vi "Execute received commands.vi"(8 "error in (no error)":errorcluster, 10 "WCM_state":bool=TRUE, 11 "Control-Client in":refnum<class "Control-Client.lvclass">) -> (0 "error out":errorcluster, 3 "Control-Client out":refnum<class "Control-Client.lvclass">)   [LabVIEW 2018, in "Control-Client.lvclass"]
uses:
  Control-Client.lvclass
  C:/Users/Sergey Denisov/Documents/REPS/TRANCON/Classes/GeneralFunctionality/GeneralFunctionality.lvclass
  dependecies/ControlsVIs/Clusters-def/Det-Reply-to-Read.ctl
  dependecies/ControlsVIs/Clusters-def/Def_signals_from_DET.ctl
  dependecies/ControlsVIs/Clusters-def/Message types.ctl
  dependecies/ControlsVIs/Clusters-def/Standard Command.ctl
  Control-Client.lvclass/Control-Client.ctl
  dependecies/ControlsVIs/Clusters-def/ProtypeCommand-CommandUnknown.ctl
  <vilib>/NI/STM/TCP/TCP Connection Info.ctl
  <vilib>/NI/STM/SubVIs/MetaDataElement.ctl
  dependecies/ControlsVIs/Clusters-def/Commands-CLIENT.ctl
  dependecies/ControlsVIs/Clusters-def/DLMovedAxis-Com.ctl
  dependecies/XControls/CellsDL/ControlDL.xctl
  dependecies/ControlsVIs/Clusters-def/OSc-Reply-Read.ctl
  dependecies/ControlsVIs/Clusters-def/CONTROL-Reply-Allconnect.ctl
  dependecies/ControlsVIs/Clusters-def/ProtypeCommand-DAQmxReply.ctl
  dependecies/ControlsVIs/Clusters-def/DAQmx-ELYSE_pulse_counter.ctl
  dependecies/ControlsVIs/Clusters-def/DAQmx-ELYSE_PumpSpeed.ctl
  controls/Gauge_pump/Gauge_pump.xctl
  dependecies/average-2Darray-SD_double.vi
  Message/Message.lvclass
  <vilib>/NI/STM/NI STM.lvlib
  Control-Server/Control-Server.lvclass
  Delay Line/DelayLine.lvclass
  DAQmxTasks/DAQmxTaskContainer_General/DAQmxTaksContainer_General.lvclass
  Oscilloscope/Oscilloscope.lvclass
  GeneralFunctionality/GeneralFunctionality.lvclass
  Detector/Detector.lvclass
panel:
  in  "?":T1
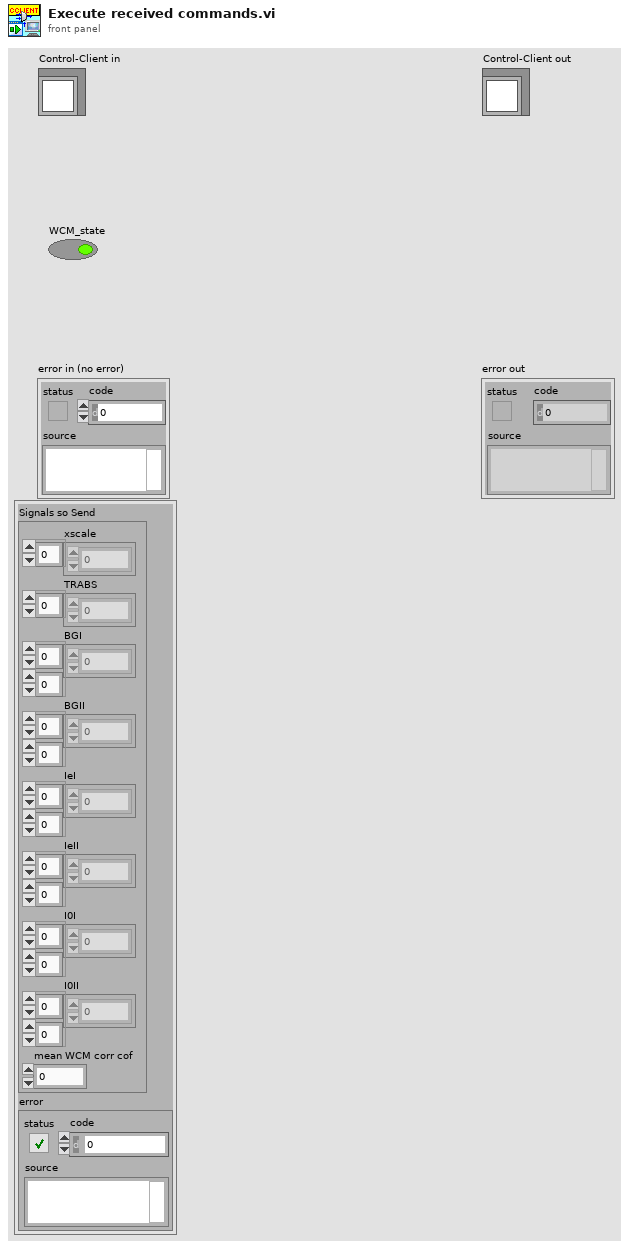
[diagram p1: front panel]
types:
  T1 = typedef "Detector.lvclass/Det-Reply-to-Read.ctl" = cluster{"Signals so Send":T2, "error":errorcluster}
  T2 = typedef "Detector.lvclass/Def_signals_from_DET.ctl" = cluster{"xscale":sgl[], "TRABS":sgl[], "BGI":sgl[][], "BGII":sgl[][], "IeI":sgl[][], "IeII":sgl[][], "I0I":sgl[][], "I0II":sgl[][], "mean WCM corr cof":dbl}
  T3 = typedef "Message types.ctl" = string
  T4 = typedef "Standard Command.ctl" = cluster{"command":string, "data":variant}
  T5 = typedef "ProtypeCommand-CommandUnknown.ctl" = cluster{"error in (no error)":errorcluster}
  T6 = typedef "Control-Client.lvclass/Commands-CLIENT.ctl" = string
  T7 = typedef "NI STM.lvlib/TCP Connection Info.ctl" = cluster{"connection ID":refnum<k5>, "meta data":T8[]}
  T8 = typedef "NI STM.lvlib/MetaDataElement.ctl" = string
  T9 = typedef "DelayLine.lvclass/DLMovedAxis-Com.ctl" = cluster{"axis":i32, "what was asked":dbl, "where is is now":dbl, "Moved":bool, "error in (no error)":errorcluster}
  T10 = typedef "Oscilloscope.lvclass/OSc-Reply-Read.ctl" = cluster{"Data":waveform(dbl)[], "Channels":u16[], "error":errorcluster}
  T11 = typedef "Control-Server.lvclass/CONTROL-Reply-Allconnect.ctl" = cluster{"On/Off":bool, "error":errorcluster}
  T12 = typedef "ProtypeCommand-DAQmxReply.ctl" = cluster{"On/Off":bool, "error out":errorcluster}
  T13 = enum8{"Enabled", "Disabled", "Disabled and Grayed Out"}
  T14 = typedef "DAQmxTaksContainer_General.lvclass/DAQmx-ELYSE_pulse_counter.ctl" = cluster{"# counts":dbl}
  T15 = cluster{"Data":dbl, "direction":bool, "start/stop":bool}
  T16 = typedef "DAQmxTaksContainer_General.lvclass/DAQmx-ELYSE_PumpSpeed.ctl" = cluster{"speed, rpm":dbl}
  T17 = typedef "Control-Client.lvclass/Controls-with-permissions_CLIENT.ctl" = cluster{"Server ON/OFF":refnum<vi>, "Detector connect":refnum<vi>, "DL connect":refnum<vi>, "DAQmx connect":refnum<vi>, "All connect":refnum<vi>, "Start measurement":refnum<vi>, "Move Crystal":refnum<vi>, "Relay key heater":refnum<vi>, "Laser Shutter":refnum<vi>, "Accelerator Shutter":refnum<vi>, "Power":refnum<vi>, "Unlock":refnum<vi>, "RT":refnum<vi>, "Faraday Cup":refnum<vi>, "Osc connect":refnum<vi>, "ELYSE pulses":refnum<vi>, "Cells":refnum<vi>, "Pump":refnum<vi>, "# par point":refnum<vi>, "Alarm":refnum<vi>, "oscilloscopeRead":refnum<vi>, "WCM_state":refnum<vi>, "ControlDL":refnum<vi>}
  T18 = typedef "graphs_TR.ctl" = cluster{"TR SC":refnum<vi>, "TR OD":refnum<vi>, "Raw data":refnum<vi>, "Raw data BG":refnum<vi>}
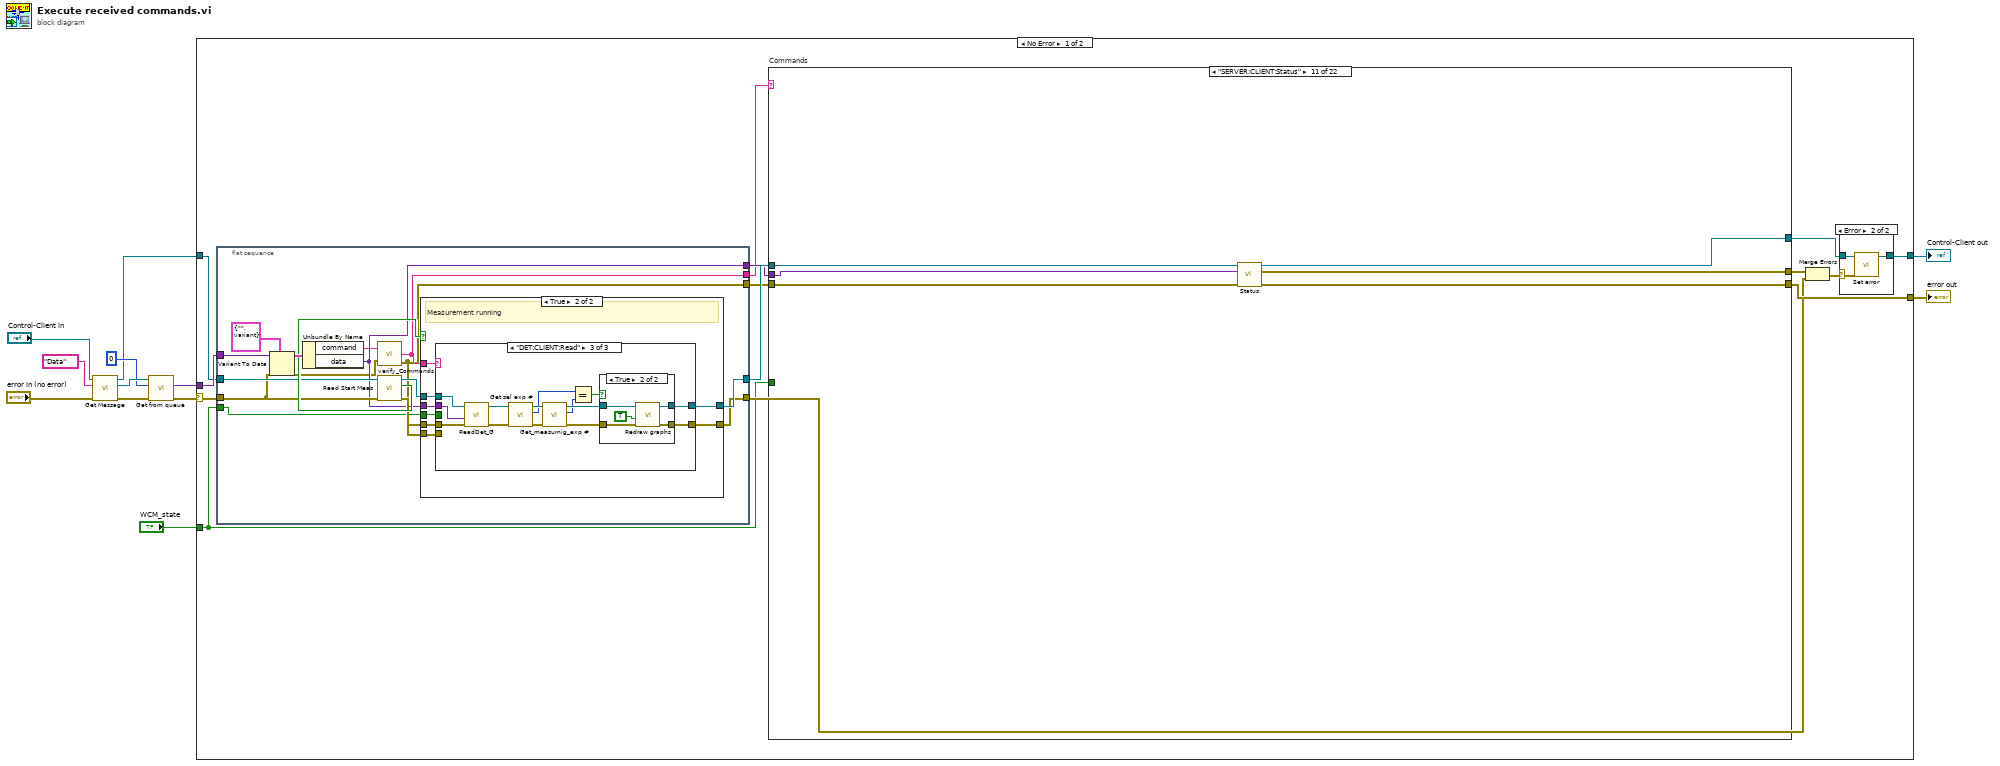
[diagram p0: block diagram]
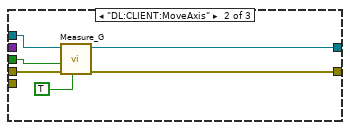
[diagram p5: hidden frame]
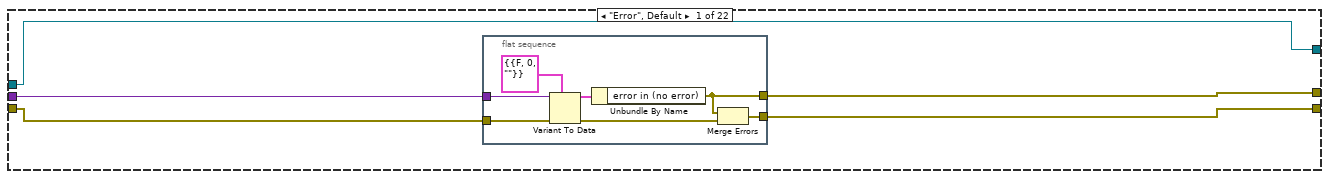
[diagram p7: hidden frame]
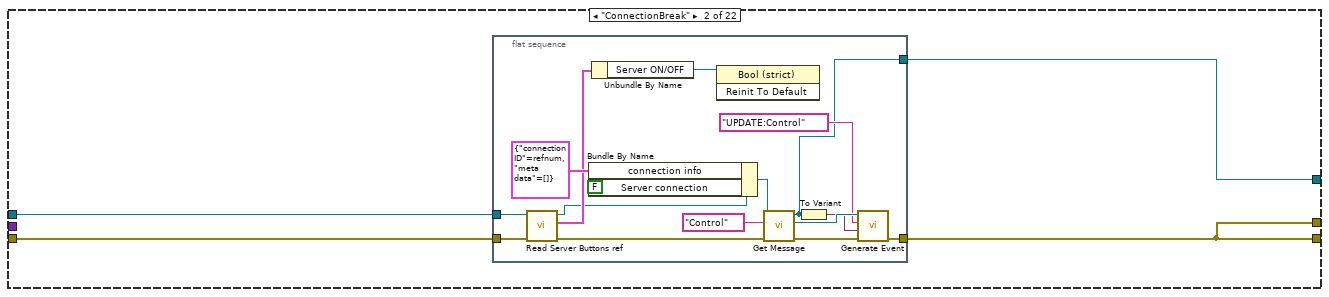
[diagram p8: hidden frame]
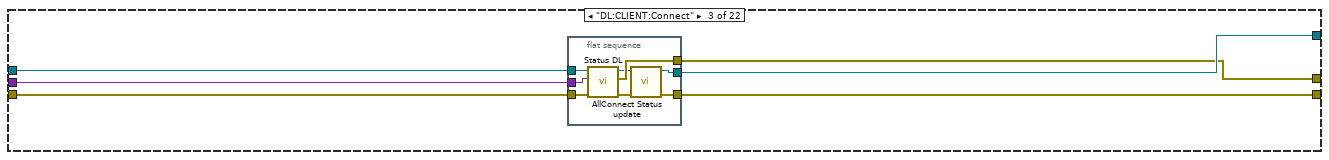
[diagram p9: hidden frame]
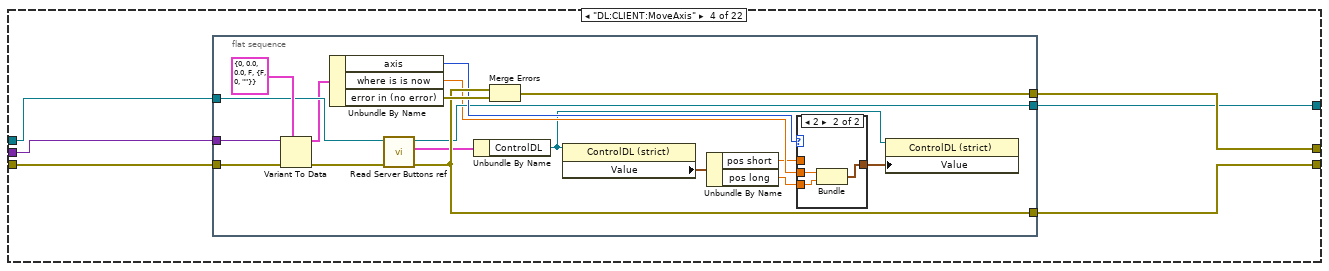
[diagram p10: hidden frame]
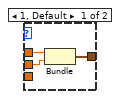
[diagram p11: hidden frame]
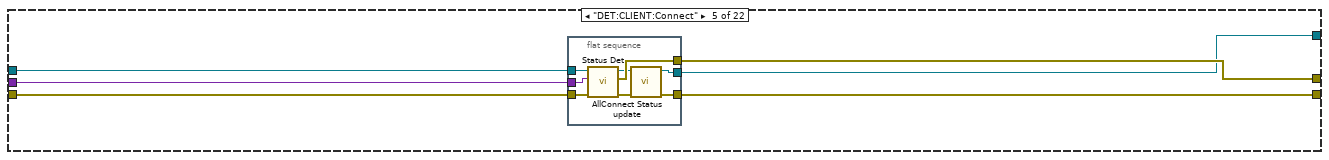
[diagram p12: hidden frame]
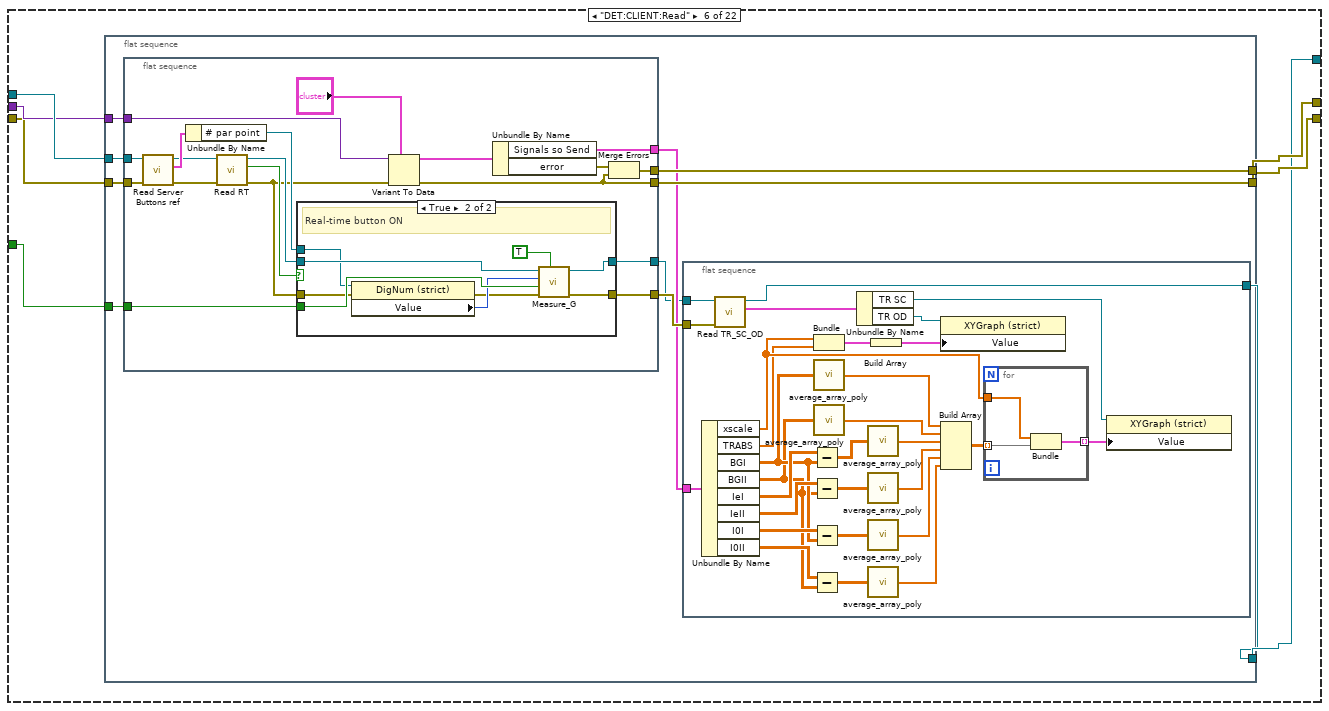
[diagram p13: hidden frame]
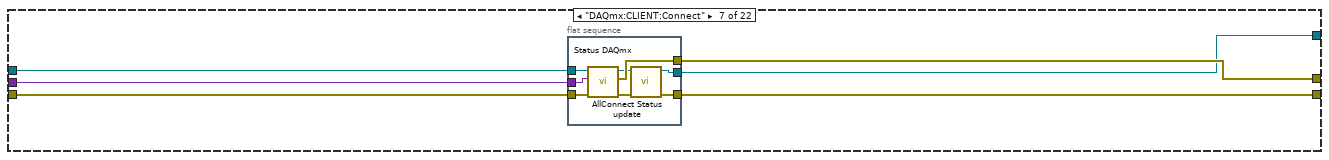
[diagram p15: hidden frame]
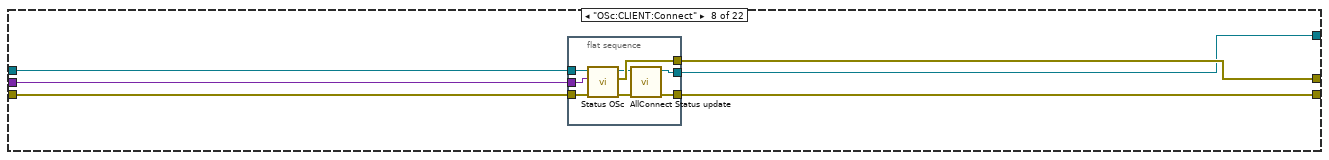
[diagram p16: hidden frame]
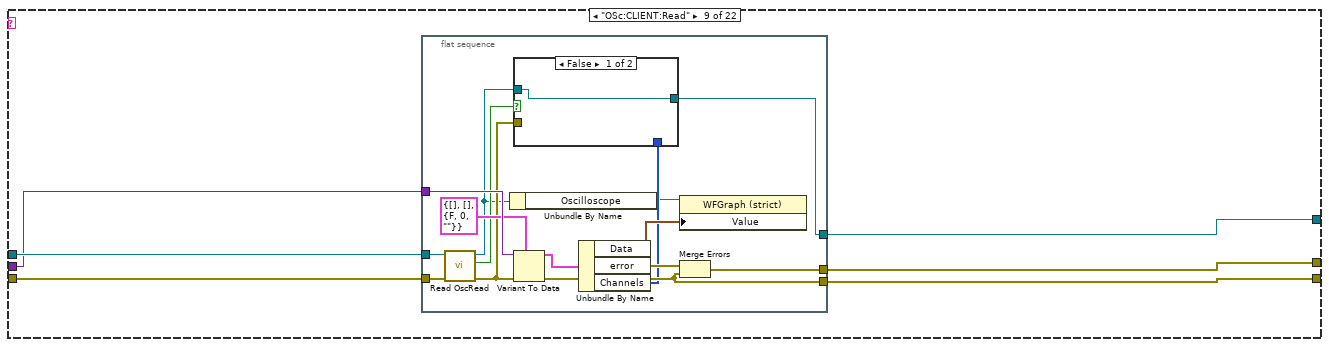
[diagram p17: hidden frame]
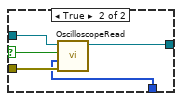
[diagram p18: hidden frame]
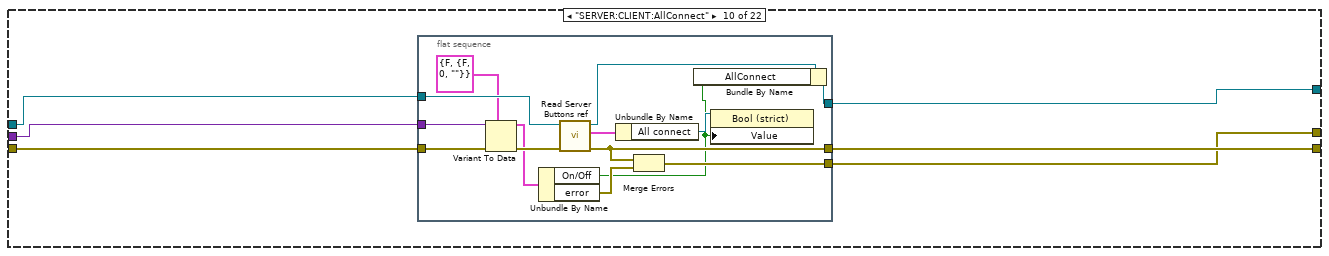
[diagram p19: hidden frame]
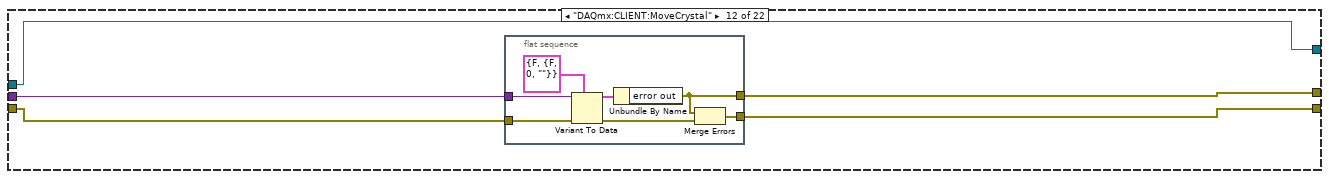
[diagram p20: hidden frame]
diagram:
  n1 = call "Get Message.vi"("error in (no error)"="error in (no error)", "Message type"=T3 "Data", "GeneralFunctionality en entrée"="Control-Client in") -> ("error out"=w6:errorcluster, "Message.lvclass"=w7:refnum<class "Message.lvclass">, "GeneralFunctionality en sortie"=w1:refnum<class "Control-Client.lvclass">)  [unwired: 6 in]
  n2 = call "Get from queue.vi"("error in (no error)"=w6, "timeout in ms (-1)"=0, "Message in"=w7) -> ("error out"=w5:errorcluster, "Data"=w4:variant)  [unwired: 5 in, 2 out]
  n3 = case shown="No Error" w5 {
    selector: w5 -> [w21 w531]
    tunnel: w4 -> [w26 _]
    tunnel: w1 -> [w22 w530]
    tunnel: [w25 w531] -> w11
    tunnel: [w23 w530] -> w9
    tunnel: "WCM_state" -> [w14 _]
    frame No Error {
      n4 = flat-sequence {
        tunnel: w26 -> [w46]
        tunnel: w22 -> [w42]
        tunnel: w21 -> [w41]
        tunnel: [w38] -> w19
        tunnel: [w37] -> w18
        tunnel: [w34] -> w17
        tunnel: [w33] -> w16
        tunnel: [w32] -> w15
        tunnel: w14 -> [w31]
        frame #0 {
          n5 = Variant To Data(error in=w41, type=T4 {"command"="", "data"=variant} ("input cluster"), Variant=w46) -> (data=w44:T4, error out=w36:errorcluster)
          n6 = Unbundle By Name(w44) -> ("command"=w35:string, "data"=w37:variant)
          n7 = call "verify_Commands.vi"("Command"=w35, "error in"=w36) -> ("Command out"=w34:string, "error out"=w33:errorcluster)  [unwired: 1 out]
          n8 = call "Read Start Meas.vi"("error in (no error)"=w41, "Control-Client in"=w42) -> ("error out"=w40:errorcluster, "Start Meas"=w43:bool, "Control-Client out"=w39:refnum<class "Control-Client.lvclass">)  [unwired: 7 in]
          n9 = case shown="True" w43 {
            tunnel: w34 -> [_ w56]
            tunnel: w40 -> [w48 w55]
            tunnel: [w48 w52] -> w32
            tunnel: w39 -> [w47 w54]
            tunnel: [w47 w53] -> w38
            tunnel: w37 -> [_ w51]
            tunnel: w33 -> [_ w50]
            tunnel: w31 -> [_ w49]
            frame False {
              # "Measurement not running"
            }
            frame True {
              # "Measurement running"
              n10 = case shown="\"DET:CLIENT:Read\"" w56 {
                tunnel: w55 -> [_ w61 w78]
                tunnel: [w57 w64 w76] -> w52
                tunnel: w54 -> [w58 w62 w77]
                tunnel: [w58 w63 w75] -> w53
                tunnel: w51 -> [_ _ w74]
                tunnel: w50 -> [w57 _ _]
                tunnel: w49 -> [_ w60 _]
                frame "Error", Default {
                }
                frame "DL:CLIENT:MoveAxis" {
                  n11 = call "Measure_G.vi"("Internal"=TRUE ("Inernal"), "error in (no error)"=w61, "WCM_correction"=w60, "Control-Client in"=w62) -> ("error out"=w64:errorcluster, "Control-Client out"=w63:refnum<class "Control-Client.lvclass">)  [unwired: 6 in]
                }
                frame "DET:CLIENT:Read" {
                  n12 = call "ReadDet_G.vi"("error in (no error)"=w78, "data"=w74, "Control-Client in"=w77) -> ("error out"=w69:errorcluster, "Control-Client out"=w72:refnum<class "Control-Client.lvclass">)  [unwired: 7 in]
                  n13 = call "Get sel exp #.vi"("error in (no error)"=w69, "Control-Client in"=w72) -> ("error out"=w70:errorcluster, "Exp sel #"=w67:i32, "Control-Client out"=w73:refnum<class "Control-Client.lvclass">)  [unwired: 7 in]
                  n14 = call "Get_measurnig_exp #.vi"("error in (no error)"=w70, "Control-Client in"=w73) -> ("error out"=w68:errorcluster, "Exp measuring #"=w66:i32, "Control-Client out"=w71:refnum<class "Control-Client.lvclass">)  [unwired: 7 in]
                  n15 = Equal?(x=w67, y=w66) -> (x = y?=w65:bool)
                  n16 = case shown="True" w65 {
                    tunnel: [w80 w85] -> w76
                    tunnel: [w79 w84] -> w75
                    tunnel: w71 -> [w79 w82]
                    tunnel: w68 -> [w80 w81]
                    frame False {
                    }
                    frame True {
                      n17 = call "Redraw graphs.vi"("error in (no error)"=w81, "Selected exp"=TRUE, "Control-Client in"=w82) -> ("error out"=w85:errorcluster, "Control-Client out"=w84:refnum<class "Control-Client.lvclass">)  [unwired: 7 in]
                    }
                  }
                }
              }
            }
          }
        }
      }
      n18 = case "Commands" shown="\"SERVER:CLIENT:Status\"" w17 {
        tunnel: w18 -> [w90 _ w123 w137 w167 w181 w260 w274 w287 w315 w335 w340 w353 w370 w389 w410 w431 w450 w467 w487 w506 w522]
        tunnel: w19 -> [w89 w99 w122 w135 w166 w182 w259 w273 w288 w314 w334 w338 w352 w372 w391 w409 w432 w451 w468 w488 w507 w523]
        tunnel: w16 -> [w87 w98 w121 w136 w165 w177 w258 w272 w283 w313 w333 w337 w351 w371 w390 w408 w433 w452 w469 w483 w502 w518]
        tunnel: [w86 w100 w119 w133 w162 w180 w255 w269 w286 w311 w331 w336 w350 w369 w386 w407 w430 w449 w466 w486 w505 w521] -> w25
        tunnel: [w89 w101 w120 w132 w163 w178 w256 w270 w284 w312 w332 w338 w348 w367 w388 w405 w428 w447 w464 w484 w503 w519] -> w24
        tunnel: [w88 w100 w118 w134 w164 w179 w257 w271 w285 w310 w330 w339 w349 w368 w387 w406 w429 w448 w465 w485 w504 w520] -> w20
        tunnel: w14 -> [_ _ _ _ _ w176 _ _ _ _ _ _ _ _ _ _ _ _ _ _ _ _]
        frame "Error", Default {
          n19 = flat-sequence {
            tunnel: w90 -> [w97]
            tunnel: [w93] -> w88
            tunnel: w87 -> [w94]
            tunnel: [w91] -> w86
            frame #0 {
              n20 = Variant To Data(error in=w94, type=T5 {"error in (no error)"={"status"=FALSE, "code"=0, "source"=""}} ("cluster"), Variant=w97) -> (data=w95:T5, error out=w92:errorcluster)
              n21 = Unbundle By Name(w95) -> ("error in (no error)"=w93:errorcluster)
              n22 = Merge Errors(w93, w92) -> (w91:errorcluster)
            }
          }
        }
        frame "ConnectionBreak" {
          n23 = flat-sequence {
            tunnel: [w102] -> w101
            tunnel: [w110] -> w100
            tunnel: w99 -> [w109]
            tunnel: w98 -> [w108]
            frame #0 {
              n24 = call "Read Server Buttons ref.vi"("error in (no error)"=w108, "Control-Client in"=w109) -> ("error out"=w107:errorcluster, "Server Buttons ref"=w106:T17, "Control-Client out"=w103:refnum<class "Control-Client.lvclass">)  [unwired: 7 in]
              n25 = Bundle By Name(cluster=w103, "connection info"=T7 {"connection ID"=refnum, "meta data"=[]}, "Server connection"=FALSE) -> (w111:refnum<class "Control-Client.lvclass">)
              n26 = Unbundle By Name(w106) -> ("Server ON/OFF"=w104:refnum<vi>)
              n27 = invoke class="Bool (strict)" method="Reinit To Default"(reference=w104) -> ()  [unwired: 2 in, 3 out]
              n28 = call "Get Message.vi"("error in (no error)"=w107, "Message type"=T3 "Control", "GeneralFunctionality en entrée"=w111) -> ("error out"=w115:errorcluster, "Message.lvclass"=w114:refnum<class "Message.lvclass">, "GeneralFunctionality en sortie"=w102:refnum<class "Control-Client.lvclass">)  [unwired: 6 in]
              n29 = To Variant(anything=w102) -> (Variant=w112:variant)
              n30 = call "Generate Event.vi"("error in (no error)"=w115, "Data"=w112, "Command"=T6 "UPDATE:Control" ("Commands-Client"), "Message en entrée"=w114) -> ("error out"=w110:errorcluster)  [unwired: 6 in, 1 out]
            }
          }
        }
        frame "DL:CLIENT:Connect" {
          n31 = flat-sequence {
            tunnel: w123 -> [w131]
            tunnel: w122 -> [w130]
            tunnel: w121 -> [w129]
            tunnel: [w126] -> w120
            tunnel: [w125] -> w119
            tunnel: [w128] -> w118
            frame #0 {
              n32 = call "Status DL.vi"("error in (no error)"=w129, "data"=w131, "Control-Client in"=w130) -> ("error out"=w124:errorcluster, "error IO"=w128:errorcluster, "Control-Client out"=w127:refnum<class "Control-Client.lvclass">)  [unwired: 6 in]
              n33 = call "AllConnect Status update.vi"("error in (no error)"=w124, "Control-Client in"=w127) -> ("error out"=w125:errorcluster, "Control-Client out"=w126:refnum<class "Control-Client.lvclass">)  [unwired: 8 in]
            }
          }
        }
        frame "DL:CLIENT:MoveAxis" {
          n34 = flat-sequence {
            tunnel: w137 -> [w155]
            tunnel: w136 -> [w154]
            tunnel: w135 -> [w151]
            tunnel: [w148] -> w134
            tunnel: [w147] -> w133
            tunnel: [w145] -> w132
            frame #0 {
              n35 = Variant To Data(error in=w154, type=T9 {"axis"=0, "what was asked"=0.0, "where is is now"=0.0, "Moved"=FALSE, "error in (no error)"={"status"=FALSE, "code"=0, "source"=""}} ("cluster"), Variant=w155) -> (data=w150:T9, error out=w152:errorcluster)
              n36 = Unbundle By Name(w150) -> ("axis"=w146:i32, "where is is now"=w144:dbl, "error in (no error)"=w149:errorcluster)
              n37 = call "Read Server Buttons ref.vi"("error in (no error)"=w152, "Control-Client in"=w151) -> ("error out"=w147:errorcluster, "Server Buttons ref"=w142:T17, "Control-Client out"=w145:refnum<class "Control-Client.lvclass">)  [unwired: 7 in]
              n38 = Unbundle By Name(w142) -> ("ControlDL"=w139:refnum<vi>)
              n39 = Merge Errors(w147, w149) -> (w148:errorcluster)
              n40 = property class="ControlDL (strict)"(reference=w139) -> ("Value"=w141:cluster{"pos short":dbl, "pos long":dbl})  [unwired: 1 in, 2 out]
              n41 = Unbundle By Name(w141) -> ("pos short"=w140:dbl, "pos long"=w138:dbl)
              n42 = case shown="2" w146 {
                tunnel: w144 -> [w158 w161]
                tunnel: [w157 w159] -> w143
                tunnel: w140 -> [w156 _]
                tunnel: w138 -> [_ w160]
                frame 1, Default {
                  n43 = Bundle("pos short"=w156, "where is is now"=w158) -> (w157:cluster{"pos short":dbl, "where is is now":dbl})  [unwired: 1 in]
                }
                frame 2 {
                  n44 = Bundle("where is is now"=w161, "pos long"=w160) -> (w159:cluster{"where is is now":dbl, "pos long":dbl})  [unwired: 1 in]
                }
              }
              n45 = property class="ControlDL (strict)"(reference=w139, "Value"=w143) -> ()  [unwired: 1 in, 2 out]
            }
          }
        }
        frame "DET:CLIENT:Connect" {
          n46 = flat-sequence {
            tunnel: w167 -> [w175]
            tunnel: w166 -> [w174]
            tunnel: w165 -> [w173]
            tunnel: [w172] -> w164
            tunnel: [w170] -> w163
            tunnel: [w168] -> w162
            frame #0 {
              n47 = call "Status Det.vi"("error in (no error)"=w173, "data"=w175, "Control-Client in"=w174) -> ("error out"=w169:errorcluster, "error IO"=w172:errorcluster, "Control-Client out"=w171:refnum<class "Control-Client.lvclass">)  [unwired: 6 in]
              n48 = call "AllConnect Status update.vi"("error in (no error)"=w169, "Control-Client in"=w171) -> ("error out"=w168:errorcluster, "Control-Client out"=w170:refnum<class "Control-Client.lvclass">)  [unwired: 8 in]
            }
          }
        }
        frame "DET:CLIENT:Read" {
          n49 = flat-sequence {
            tunnel: w182 -> [w189]
            tunnel: w181 -> [w192]
            tunnel: [w191] -> w180
            tunnel: [w190] -> w179
            tunnel: [w183] -> w178
            tunnel: w177 -> [w188]
            tunnel: w176 -> [w185]
            frame #0 {
              n50 = flat-sequence {
                tunnel: w192 -> [w211]
                tunnel: [w210] -> w191
                tunnel: [w209] -> w190
                tunnel: w189 -> [w205]
                tunnel: w188 -> [w199]
                tunnel: [w195] -> w187
                tunnel: [w201] -> w186
                tunnel: w185 -> [w200]
                tunnel: [w197] -> w184
                frame #0 {
                  n51 = call "Read Server Buttons ref.vi"("error in (no error)"=w199, "Control-Client in"=w205) -> ("error out"=w193:errorcluster, "Server Buttons ref"=w204:T17, "Control-Client out"=w194:refnum<class "Control-Client.lvclass">)  [unwired: 7 in]
                  n52 = Unbundle By Name(w204) -> ("# par point"=w203:refnum<vi>)
                  n53 = call "Read RT.vi"("error in (no error)"=w193, "Control-Client in"=w194) -> ("error out"=w196:errorcluster, "RT"=w202:bool, "Control-Client out"=w198:refnum<class "Control-Client.lvclass">)  [unwired: 7 in]
                  n54 = case shown="True" w202 {
                    tunnel: w198 -> [w213 w222]
                    tunnel: w196 -> [w212 w217]
                    tunnel: w203 -> [_ w219]
                    tunnel: w200 -> [_ w221]
                    tunnel: [w213 w215] -> w197
                    tunnel: [w212 w214] -> w195
                    frame False {
                    }
                    frame True {
                      # "Real-time button ON"
                      n55 = property class="DigNum (strict)"(reference=w219, error in=w217) -> (error out=w216:errorcluster, "Value"=w218:i32)  [unwired: 1 out]
                      n56 = call "Measure_G.vi"("All"=TRUE, "error in (no error)"=w216, "WCM_correction"=w221, "# scans"=w218, "Control-Client in"=w222) -> ("error out"=w214:errorcluster, "Control-Client out"=w215:refnum<class "Control-Client.lvclass">)  [unwired: 5 in]
                    }
                  }
                  n57 = Variant To Data(error in=w196, type="?", Variant=w211) -> (data=w207:T1, error out=w210:errorcluster)
                  n58 = Unbundle By Name(w207) -> ("Signals so Send"=w201:T2, "error"=w206:errorcluster)
                  n59 = Merge Errors(w206, w210) -> (w209:errorcluster)
                }
              }
              n60 = flat-sequence {
                tunnel: w187 -> [w236]
                tunnel: w186 -> [w246]
                tunnel: w184 -> [w234]
                tunnel: [w233] -> w183
                frame #0 {
                  n61 = Unbundle By Name(w246) -> ("xscale"=w248:sgl[], "TRABS"=w247:sgl[], "BGI"=w224:sgl[][], "BGII"=w223:sgl[][], "IeI"=w232:sgl[][], "IeII"=w230:sgl[][], "I0I"=w228:sgl[][], "I0II"=w225:sgl[][])
                  n62 = call "Read TR_SC_OD.vi"("error in (no error)"=w236, "Control-Client en entrée"=w234) -> ("TR_SC_OD"=w235:T18, "Control-Client en sortie"=w233:refnum<class "Control-Client.lvclass">)  [unwired: 7 in, 1 out]
                  n63 = Subtract(x=w232, y=w224) -> (x-y=w231:sgl[][])
                  n64 = Subtract(x=w230, y=w223) -> (x-y=w229:sgl[][])
                  n65 = Subtract(x=w228, y=w224) -> (x-y=w227:sgl[][])
                  n66 = Subtract(x=w225, y=w223) -> (x-y=w226:sgl[][])
                  n67 = Bundle("xscale"=w248, "TRABS"=w247) -> (w249:cluster{"xscale":sgl[], "TRABS":sgl[]})  [unwired: 1 in]
                  n68 = call-poly "average_array_poly.vi"("2D array"=w224) -> ("out array"=w242:dbl[])
                  n69 = call-poly "average_array_poly.vi"("2D array"=w223) -> ("out array"=w241:dbl[])
                  n70 = Unbundle By Name(w235) -> ("TR SC"=w251:refnum<vi>, "TR OD"=w250:refnum<vi>)
                  n71 = call-poly "average_array_poly.vi"("2D array"=w231) -> ("out array"=w240:dbl[])
                  n72 = call-poly "average_array_poly.vi"("2D array"=w229) -> ("out array"=w239:dbl[])
                  n73 = call-poly "average_array_poly.vi"("2D array"=w227) -> ("out array"=w238:dbl[])
                  n74 = call-poly "average_array_poly.vi"("2D array"=w226) -> ("out array"=w237:dbl[])
                  n75 = Build Array(w249) -> (w243:cluster{"xscale":sgl[], "TRABS":sgl[]}[])
                  n76 = property class="XYGraph (strict)"(reference=w250, "Value"=w243) -> ()  [unwired: 1 in, 2 out]
                  n77 = Build Array(w242, w241, w240, w239, w238, w237) -> (w245:dbl[][])
                  n78 = for {
                    tunnel: [w254] -> w244 mode=indexing
                    tunnel: w248 -> [w253]
                    tunnel: w245 -> [w252] mode=indexing
                    n79 = Bundle("xscale"=w253, w252) -> (w254:cluster{"xscale":sgl[], dbl[]})  [unwired: 1 in]
                  }
                  n80 = property class="XYGraph (strict)"(reference=w251, "Value"=w244) -> ()  [unwired: 1 in, 2 out]
                }
              }
            }
          }
        }
        frame "DAQmx:CLIENT:Connect" {
          n81 = flat-sequence {
            tunnel: w260 -> [w268]
            tunnel: w259 -> [w267]
            tunnel: w258 -> [w266]
            tunnel: [w265] -> w257
            tunnel: [w262] -> w256
            tunnel: [w261] -> w255
            frame #0 {
              n82 = call "Status DAQmx.vi"("error in (no error)"=w266, "data"=w268, "Control-Client in"=w267) -> ("error out"=w263:errorcluster, "error IO"=w265:errorcluster, "Control-Client out"=w264:refnum<class "Control-Client.lvclass">)  [unwired: 6 in]
              n83 = call "AllConnect Status update.vi"("error in (no error)"=w263, "Control-Client in"=w264) -> ("error out"=w261:errorcluster, "Control-Client out"=w262:refnum<class "Control-Client.lvclass">)  [unwired: 8 in]
            }
          }
        }
        frame "OSc:CLIENT:Connect" {
          n84 = flat-sequence {
            tunnel: w274 -> [w282]
            tunnel: w273 -> [w281]
            tunnel: w272 -> [w280]
            tunnel: [w279] -> w271
            tunnel: [w276] -> w270
            tunnel: [w275] -> w269
            frame #0 {
              n85 = call "Status OSc.vi"("error in (no error)"=w280, "data"=w282, "Control-Client in"=w281) -> ("error out"=w277:errorcluster, "error IO"=w279:errorcluster, "Control-Client out"=w278:refnum<class "Control-Client.lvclass">)  [unwired: 6 in]
              n86 = call "AllConnect Status update.vi"("error in (no error)"=w277, "Control-Client in"=w278) -> ("error out"=w275:errorcluster, "Control-Client out"=w276:refnum<class "Control-Client.lvclass">)  [unwired: 8 in]
            }
          }
        }
        frame "OSc:CLIENT:Read" {
          n87 = flat-sequence {
            tunnel: w288 -> [w296]
            tunnel: w287 -> [w303]
            tunnel: [w301] -> w286
            tunnel: [w300] -> w285
            tunnel: [w289] -> w284
            tunnel: w283 -> [w297]
            frame #0 {
              n88 = call-dynamic "Read OscRead.vi"("error in (no error)"=w297, "Control-Client in"=w296) -> ("error out"=w294:errorcluster, "OscRead"=w295:bool, "Control-Client out"=w291:refnum<class "Control-Client.lvclass">)  [unwired: 7 in]
              n89 = Unbundle By Name(w291) -> ("Oscilloscope"=w290:refnum<vi>)
              n90 = Variant To Data(error in=w294, type=T10 {"Data"=[], "Channels"=[], "error"={"status"=FALSE, "code"=0, "source"=""}} ("Cluster"), Variant=w303) -> (data=w298:T10, error out=w301:errorcluster)
              n91 = Unbundle By Name(w298) -> ("Data"=w293:waveform(dbl)[], "error"=w302:errorcluster, "Channels"=w292:u16[])
              n92 = case shown="False" w295 {
                selector: w295 -> [_ w309]
                tunnel: w291 -> [w304 w308]
                tunnel: w294 -> [_ w307]
                tunnel: w292 -> [_ w306]
                tunnel: [w304 w305] -> w289
                frame False {
                }
                frame True {
                  n93 = call "OscilloscopeRead.vi"("error in (no error)"=w307, "channelsOsc"=w306, "ON/OFF"=w309, "Control-Client in"=w308) -> ("Control-Client out"=w305:refnum<class "Control-Client.lvclass">)  [unwired: 6 in, 1 out]
                }
              }
              n94 = property class="WFGraph (strict)"(reference=w290, "Value"=w293) -> ()  [unwired: 1 in, 2 out]
              n95 = Merge Errors(w302, w301) -> (w300:errorcluster)
            }
          }
        }
        frame "SERVER:CLIENT:AllConnect" {
          n96 = flat-sequence {
            tunnel: w315 -> [w329]
            tunnel: w314 -> [w328]
            tunnel: w313 -> [w326]
            tunnel: [w318] -> w312
            tunnel: [w320] -> w311
            tunnel: [w319] -> w310
            frame #0 {
              n97 = Variant To Data(error in=w326, type=T11 {"On/Off"=FALSE, "error"={"status"=FALSE, "code"=0, "source"=""}} ("output cluster"), Variant=w329) -> (data=w322:T11, error out=w327:errorcluster)
              n98 = Unbundle By Name(w322) -> ("On/Off"=w316:bool, "error"=w321:errorcluster)
              n99 = call "Read Server Buttons ref.vi"("error in (no error)"=w327, "Control-Client in"=w328) -> ("error out"=w320:errorcluster, "Server Buttons ref"=w325:T17, "Control-Client out"=w317:refnum<class "Control-Client.lvclass">)  [unwired: 7 in]
              n100 = Unbundle By Name(w325) -> ("All connect"=w324:refnum<vi>)
              n101 = Merge Errors(w320, w321) -> (w319:errorcluster)
              n102 = Bundle By Name(cluster=w317, "AllConnect"=w316) -> (w318:refnum<class "Control-Client.lvclass">)
              n103 = property class="Bool (strict)"(reference=w324, "Value"=w316) -> ()  [unwired: 1 in, 2 out]
            }
          }
        }
        frame "SERVER:CLIENT:Status" {
          n104 = call "Status.vi"("error in (no error)"=w333, "data"=w335, "Control-Client in"=w334) -> ("error out"=w331:errorcluster, "error IO"=w330:errorcluster, "Control-Client out"=w332:refnum<class "Control-Client.lvclass">)  [unwired: 6 in]
        }
        frame "DAQmx:CLIENT:MoveCrystal" {
          n105 = flat-sequence {
            tunnel: w340 -> [w347]
            tunnel: [w341] -> w339
            tunnel: w337 -> [w344]
            tunnel: [w342] -> w336
            frame #0 {
              n106 = Variant To Data(error in=w344, type=T12 {"On/Off"=FALSE, "error out"={"status"=FALSE, "code"=0, "source"=""}} ("output cluster"), Variant=w347) -> (data=w345:T12, error out=w343:errorcluster)
              n107 = Unbundle By Name(w345) -> ("error out"=w341:errorcluster)
              n108 = Merge Errors(w341, w343) -> (w342:errorcluster)
            }
          }
        }
        frame "DAQmx:CLIENT:LaserShutter" {
          n109 = flat-sequence {
            tunnel: w353 -> [w366]
            tunnel: w352 -> [w365]
            tunnel: w351 -> [w364]
            tunnel: [w362] -> w350
            tunnel: [w361] -> w349
            tunnel: [w354] -> w348
            frame #0 {
              n110 = call "Read Server Buttons ref.vi"("error in (no error)"=w364, "Control-Client in"=w365) -> ("error out"=w355:errorcluster, "Server Buttons ref"=w360:T17, "Control-Client out"=w354:refnum<class "Control-Client.lvclass">)  [unwired: 7 in]
              n111 = Variant To Data(error in=w355, type=T12 {"On/Off"=FALSE, "error out"={"status"=FALSE, "code"=0, "source"=""}} ("output cluster"), Variant=w366) -> (data=w357:T12, error out=w362:errorcluster)
              n112 = Unbundle By Name(w360) -> ("Laser Shutter"=w359:refnum<vi>)
              n113 = Unbundle By Name(w357) -> ("On/Off"=w356:bool, "error out"=w363:errorcluster)
              n114 = property class="Bool (strict)"(reference=w359, "Value"=w356) -> ()  [unwired: 1 in, 2 out]
              n115 = Merge Errors(w363, w362) -> (w361:errorcluster)
            }
          }
        }
        frame "DAQmx:CLIENT:AcceleratorShutter" {
          n116 = flat-sequence {
            tunnel: w372 -> [w385]
            tunnel: w371 -> [w384]
            tunnel: w370 -> [w383]
            tunnel: [w381] -> w369
            tunnel: [w380] -> w368
            tunnel: [w373] -> w367
            frame #0 {
              n117 = call "Read Server Buttons ref.vi"("error in (no error)"=w384, "Control-Client in"=w385) -> ("error out"=w374:errorcluster, "Server Buttons ref"=w379:T17, "Control-Client out"=w373:refnum<class "Control-Client.lvclass">)  [unwired: 7 in]
              n118 = Variant To Data(error in=w374, type=T12 {"On/Off"=FALSE, "error out"={"status"=FALSE, "code"=0, "source"=""}} ("output cluster"), Variant=w383) -> (data=w376:T12, error out=w381:errorcluster)
              n119 = Unbundle By Name(w379) -> ("Accelerator Shutter"=w378:refnum<vi>)
              n120 = Unbundle By Name(w376) -> ("On/Off"=w375:bool, "error out"=w382:errorcluster)
              n121 = property class="Bool (strict)"(reference=w378, "Value"=w375) -> ()  [unwired: 1 in, 2 out]
              n122 = Merge Errors(w382, w381) -> (w380:errorcluster)
            }
          }
        }
        frame "DAQmx:CLIENT:FaradayCup" {
          n123 = flat-sequence {
            tunnel: w391 -> [w404]
            tunnel: w390 -> [w403]
            tunnel: w389 -> [w402]
            tunnel: [w400] -> w386
            tunnel: [w399] -> w387
            tunnel: [w392] -> w388
            frame #0 {
              n124 = call "Read Server Buttons ref.vi"("error in (no error)"=w403, "Control-Client in"=w404) -> ("error out"=w393:errorcluster, "Server Buttons ref"=w398:T17, "Control-Client out"=w392:refnum<class "Control-Client.lvclass">)  [unwired: 7 in]
              n125 = Variant To Data(error in=w393, type=T12 {"On/Off"=FALSE, "error out"={"status"=FALSE, "code"=0, "source"=""}} ("output cluster"), Variant=w402) -> (data=w395:T12, error out=w400:errorcluster)
              n126 = Unbundle By Name(w398) -> ("Faraday Cup"=w397:refnum<vi>)
              n127 = Unbundle By Name(w395) -> ("On/Off"=w394:bool, "error out"=w401:errorcluster)
              n128 = property class="Bool (strict)"(reference=w397, "Value"=w394) -> ()  [unwired: 1 in, 2 out]
              n129 = Merge Errors(w401, w400) -> (w399:errorcluster)
            }
          }
        }
        frame "DAQmx:CLIENT:RelayKeyHeater" {
          n130 = flat-sequence {
            tunnel: w410 -> [w425]
            tunnel: w409 -> [w424]
            tunnel: w408 -> [w423]
            tunnel: [w422] -> w407
            tunnel: [w420] -> w406
            tunnel: [w411] -> w405
            frame #0 {
              n131 = call "Read Server Buttons ref.vi"("error in (no error)"=w423, "Control-Client in"=w424) -> ("error out"=w412:errorcluster, "Server Buttons ref"=w419:T17, "Control-Client out"=w411:refnum<class "Control-Client.lvclass">)  [unwired: 7 in]
              n132 = Variant To Data(error in=w412, type=T12 {"On/Off"=FALSE, "error out"={"status"=FALSE, "code"=0, "source"=""}} ("output cluster"), Variant=w425) -> (data=w416:T12, error out=w422:errorcluster)
              n133 = Unbundle By Name(w419) -> ("Relay key heater"=w418:refnum<vi>, "Alarm"=w414:refnum<vi>)
              n134 = Unbundle By Name(w416) -> ("On/Off"=w415:bool, "error out"=w421:errorcluster)
              n135 = property class="Bool (strict)"(reference=w418, "Value"=w415) -> ()  [unwired: 1 in, 2 out]
              n136 = case shown="True" w415 {
                tunnel: w414 -> [_ _]
                tunnel: [T13."Disabled and Grayed Out" ("Disabled") T13."Enabled" ("Disabled")] -> w413
                frame False {
                }
                frame True {
                }
              }
              n137 = Merge Errors(w422, w421) -> (w420:errorcluster)
              n138 = property class="Bool (strict)"(reference=w414, "DisabledEnum"=w413) -> ()  [unwired: 1 in, 2 out]
            }
          }
        }
        frame "DAQmx:CLIENT:HeaterAlarm" {
          n139 = flat-sequence {
            tunnel: w433 -> [w446]
            tunnel: w432 -> [w445]
            tunnel: w431 -> [w444]
            tunnel: [w443] -> w430
            tunnel: [w442] -> w429
            tunnel: [w437] -> w428
            frame #0 {
              n140 = call "Read Server Buttons ref.vi"("error in (no error)"=w446, "Control-Client in"=w445) -> ("error out"=w438:errorcluster, "Server Buttons ref"=w441:T17, "Control-Client out"=w437:refnum<class "Control-Client.lvclass">)  [unwired: 7 in]
              n141 = Variant To Data(error in=w438, type=T12 {"On/Off"=FALSE, "error out"={"status"=FALSE, "code"=0, "source"=""}} ("output cluster"), Variant=w444) -> (data=w439:T12, error out=w443:errorcluster)
              n142 = Unbundle By Name(w441) -> ("Alarm"=w436:refnum<vi>)
              n143 = Unbundle By Name(w439) -> ("On/Off"=w435:bool, "error out"=w434:errorcluster)
              n144 = property class="Bool (strict)"(reference=w436, "Blinking"=w435) -> ()  [unwired: 1 in, 2 out]
              n145 = property class="Bool (strict)"(reference=w436, "Value"=w435) -> ()  [unwired: 1 in, 2 out]
              n146 = Merge Errors(w434, w443) -> (w442:errorcluster)
            }
          }
        }
        frame "DAQmx:CLIENT:ELYSE_pulse_counter" {
          n147 = flat-sequence {
            tunnel: w452 -> [w463]
            tunnel: w451 -> [w462]
            tunnel: w450 -> [w461]
            tunnel: [w454] -> w449
            tunnel: [w454] -> w448
            tunnel: [w456] -> w447
            frame #0 {
              n148 = call "Read Server Buttons ref.vi"("error in (no error)"=w463, "Control-Client in"=w462) -> ("error out"=w457:errorcluster, "Server Buttons ref"=w460:T17, "Control-Client out"=w456:refnum<class "Control-Client.lvclass">)  [unwired: 7 in]
              n149 = Variant To Data(error in=w457, type=T14 {"# counts"=0.0} ("ELYSE pulses counter"), Variant=w461) -> (data=w458:T14, error out=w454:errorcluster)
              n150 = Unbundle By Name(w460) -> ("ELYSE pulses"=w455:refnum<vi>)
              n151 = Unbundle By Name(w458) -> ("# counts"=w453:dbl)
              n152 = property class="DigNum (strict)"(reference=w455, "Value"=w453) -> ()  [unwired: 1 in, 2 out]
            }
          }
        }
        frame "DAQmx:CLIENT:PumpSpeed" {
          n153 = flat-sequence {
            tunnel: w469 -> [w482]
            tunnel: w468 -> [w481]
            tunnel: w467 -> [w480]
            tunnel: [w473] -> w466
            tunnel: [w473] -> w465
            tunnel: [w475] -> w464
            frame #0 {
              n154 = call "Read Server Buttons ref.vi"("error in (no error)"=w482, "Control-Client in"=w481) -> ("error out"=w476:errorcluster, "Server Buttons ref"=w479:T17, "Control-Client out"=w475:refnum<class "Control-Client.lvclass">)  [unwired: 7 in]
              n155 = Variant To Data(error in=w476, type=T16 {"speed, rpm"=0.0} ("PumpSpeed"), Variant=w480) -> (data=w477:T16, error out=w473:errorcluster)
              n156 = Unbundle By Name(w477) -> ("speed, rpm"=w470:dbl)
              n157 = Unbundle By Name(w479) -> ("Pump"=w474:refnum<vi>)
              n158 = Bundle By Name(cluster=T15 {"Data"=0.0, "direction"=FALSE, "start/stop"=FALSE} ("Value"), "Data"=w470) -> (w471:T15)
              n159 = property class="Gauge_pump (strict)"(reference=w474, "Value"=w471) -> ()  [unwired: 1 in, 2 out]
            }
          }
        }
        frame "DAQmx:CLIENT:PowerStatus" {
          n160 = flat-sequence {
            tunnel: w483 -> [_]
            tunnel: w488 -> [w494]
            tunnel: w487 -> [w501]
            tunnel: [w499] -> w486
            tunnel: [w498] -> w485
            tunnel: [w495] -> w484
            tunnel: w483 -> [w493]
            frame #0 {
              n161 = call "Read Server Buttons ref.vi"("error in (no error)"=w493, "Control-Client in"=w494) -> ("error out"=w492:errorcluster, "Control-Client out"=w491:refnum<class "Control-Client.lvclass">)  [unwired: 7 in, 1 out]
              n162 = Variant To Data(error in=w493, type=T12 {"On/Off"=FALSE, "error out"={"status"=FALSE, "code"=0, "source"=""}} ("output cluster"), Variant=w501) -> (data=w496:T12, error out=w499:errorcluster)
              n163 = Unbundle By Name(w491) -> ("Power"=w490:refnum<vi>)
              n164 = Unbundle By Name(w496) -> ("On/Off"=w489:bool, "error out"=w500:errorcluster)
              n165 = Bundle By Name(cluster=w491, "Power"=w489) -> (w495:refnum<class "Control-Client.lvclass">)
              n166 = property class="Bool (strict)"(reference=w490, "Value"=w489) -> ()  [unwired: 1 in, 2 out]
              n167 = Merge Errors(w492, w500, w499) -> (w498:errorcluster)
            }
          }
        }
        frame "DAQmx:CLIENT:FaradayCupStatus" {
          n168 = flat-sequence {
            tunnel: w502 -> [_]
            tunnel: w507 -> [w509]
            tunnel: w506 -> [w517]
            tunnel: [w515] -> w505
            tunnel: [w514] -> w504
            tunnel: [w510] -> w503
            tunnel: w502 -> [w508]
            frame #0 {
              n169 = Variant To Data(error in=w508, type=T12 {"On/Off"=FALSE, "error out"={"status"=FALSE, "code"=0, "source"=""}} ("output cluster"), Variant=w517) -> (data=w512:T12, error out=w515:errorcluster)
              n170 = Unbundle By Name(w512) -> ("On/Off"=w511:bool, "error out"=w516:errorcluster)
              n171 = Bundle By Name(cluster=w509, "FardayCup"=w511) -> (w510:refnum<class "Control-Client.lvclass">)
              n172 = Merge Errors(w516, w515) -> (w514:errorcluster)
            }
          }
        }
        frame "DAQmx:CLIENT:Status" {
          n173 = flat-sequence {
            tunnel: w523 -> [w526]
            tunnel: w522 -> [w527]
            tunnel: [w528] -> w521
            tunnel: [w524] -> w520
            tunnel: [w525] -> w519
            tunnel: w518 -> [w529]
            frame #0 {
              n174 = call "Status DAQmx.vi"("error in (no error)"=w529, "data"=w527, "Control-Client in"=w526) -> ("error out"=w528:errorcluster, "error IO"=w524:errorcluster, "Control-Client out"=w525:refnum<class "Control-Client.lvclass">)  [unwired: 6 in]
            }
          }
        }
      }
      n175 = Merge Errors(w20, w15) -> (w13:errorcluster)
      n176 = case shown="Error" w13 {
        selector: w13 -> [_ w28]
        tunnel: w24 -> [w27 w30]
        tunnel: [w27 w29] -> w23
        frame No Error {
        }
        frame Error {
          n177 = call "Set error.vi"("error in (no error)"=w28, "Control-Client in"=w30) -> ("Control-Client out"=w29:refnum<class "Control-Client.lvclass">)  [unwired: 8 in, 1 out]
        }
      }
    }
    frame Error {
    }
  }
  "error out" <- w11
  "Control-Client out" <- w9
